vi "main.vi"() -> ()   [LabVIEW 2018]
panel:
  in  "address":string="192.168.1.10"
  in  "Read 2":bool
  in  "element":u8
  out "Array 4":u8[](array[numeric]) format="%x"
  in  "Read addr":u8 format="%x"
  in  "dummy":u8 format="%x"
  in  "write data":u8 format="%x"
  in  "write addr":u8
  in  "Write":bool
  in  "stop":bool
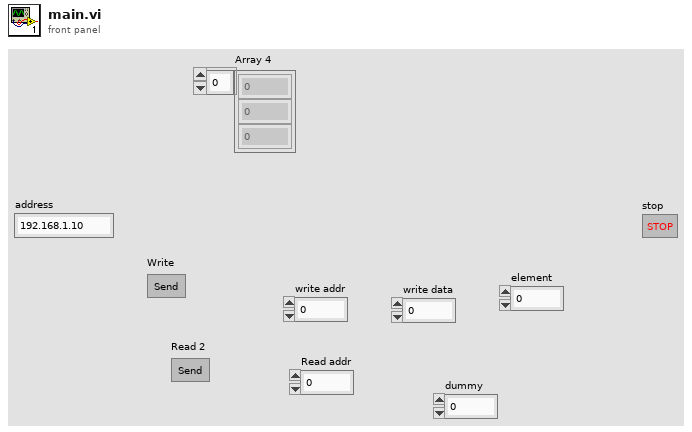
[diagram p1: front panel]
types:
  T1 = cluster{"Numeric":u8, "Numeric 2":u8, "Numeric 3":u8, u8[]}
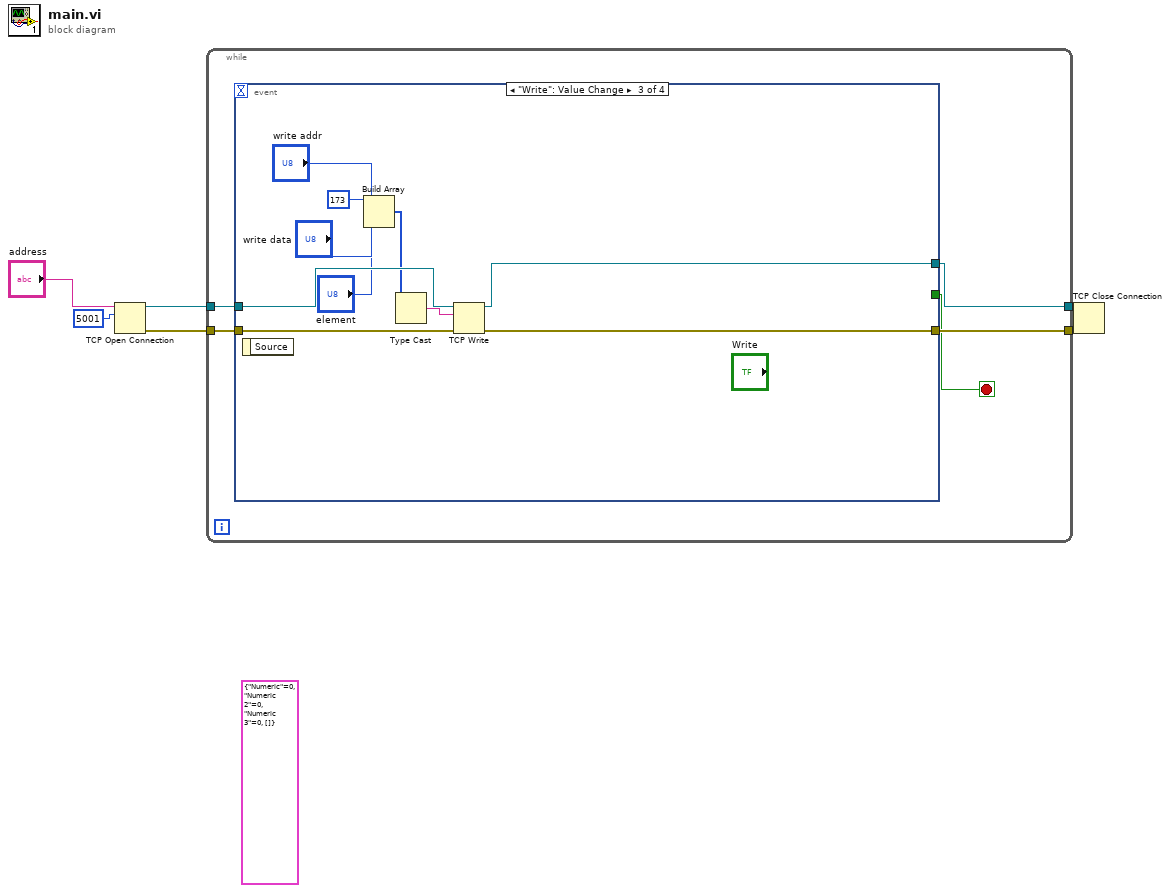
[diagram p0: block diagram]
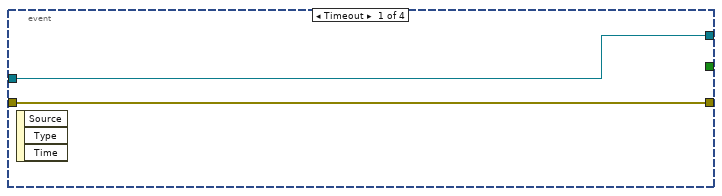
[diagram p2: hidden frame]
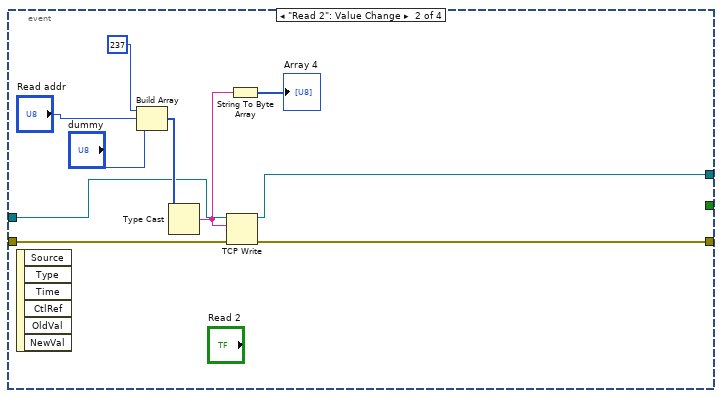
[diagram p3: hidden frame]
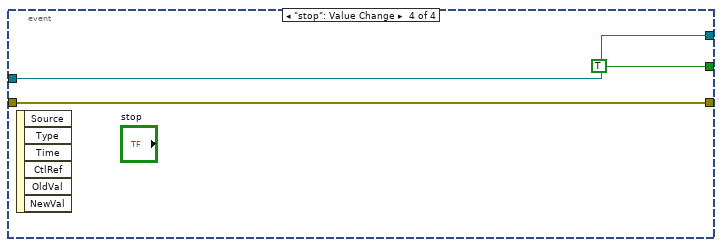
[diagram p4: hidden frame]
diagram:
  (unwired) T1 {"Numeric"=0, "Numeric 2"=0, "Numeric 3"=0, []} ("Cluster")
  n1 = TCP Open Connection(address="address", remote port or service name=u16 5001) -> (connection ID=w6:refnum<k5>, error out=w5:errorcluster)  [unwired: 3 in]
  n2 = while {
    tunnel: w5 -> [w10]
    tunnel: [w9] -> w4
    tunnel: w6 -> [w11]
    tunnel: [w8] -> w1
    stop <- w7 stop-if-true
    n3 = event shown="[2] \"Write\": Value Change" {
      selector: _ -> [_ _ _ _]
      dyn-events: _ -> [_ _ _ _]
      timeout: _ -> [_ _ _ _]
      tunnel: [_ _ _ TRUE] -> w7
      tunnel: w11 -> [w13 w17 w33 w35]
      tunnel: w10 -> [w12 w16 w32 w34]
      tunnel: [w13 w15 w25 w35] -> w8
      tunnel: [w12 w14 w24 w34] -> w9
      event Timeout {
        n4 = event-data() -> ()  [unwired: 1 in, 3 out]
      }
      event "Read 2": Value Change {
        n5 = event-data() -> ()  [unwired: 1 in, 6 out]
        n6 = Build Array(u8 237, "Read addr", "dummy") -> (w20:u8[])
        n7 = Type Cast(x=w20) -> (*(type *) &x=w23:string)  [unwired: 1 in]
        n8 = TCP Write(connection ID=w17, data in=w23, error in (no error)=w16) -> (connection ID out=w15:refnum<k5>, error out=w14:errorcluster)  [unwired: 1 in, 1 out]
        n9 = String To Byte Array(string=w23) -> (unsigned byte array=→"Array 4":u8[])
      }
      event "Write": Value Change {
        n10 = event-data() -> ()  [unwired: 1 in, 1 out]
        n11 = Build Array(u8 173, "write addr", "write data", "element") -> (w28:u8[])
        n12 = Type Cast(x=w28) -> (*(type *) &x=w31:string)  [unwired: 1 in]
        n13 = TCP Write(connection ID=w33, data in=w31, error in (no error)=w32) -> (connection ID out=w25:refnum<k5>, error out=w24:errorcluster)  [unwired: 1 in, 1 out]
      }
      event "stop": Value Change {
        n14 = event-data() -> ()  [unwired: 1 in, 6 out]
      }
    }
  }
  n15 = TCP Close Connection(connection ID=w1, error in (no error)=w4) -> ()  [unwired: 1 in, 2 out]
